vi "nD Nonlinear System Single Solution (Formula).vi"(7 "accuracy":dbl=1e-08 format="%0.2e", 8 "F(X)":string[](array[string]), 9 "X":string[](array[string]), 10 "Start":dbl[](array[numeric]) format="%0.2f", 11 "h":dbl=1e-08 format="%0.2e") -> (0 "error":i32, 1 "ticks":u32, 2 "f(Zeroes)":dbl[](array[numeric]) format="%0.2f", 3 "Zeroes":dbl[](array[numeric]) format="%0.2f")   [LabVIEW 2020, in "NI_Gmath.lvlib"]
doc: "Determines the solutions of nonlinear systems of equations in n dimensions beginning with a starting point in n dimensions. You must manually select the polymorphic instance to use."
uses:
  NI_Gmath.lvlib
  NI_AALBase.lvlib
panel:
  out "error message":string
  out "error text":string[](array[string])
  out "error code":i32[](array[numeric])
  # "Example:\n\n accuracy: 1E-8 \n h: 1E-8 \n Start: 1.0 and 0.0\n X: x and y\n F(X): sin(x+y) and cos(x-y)"
  # "error information"
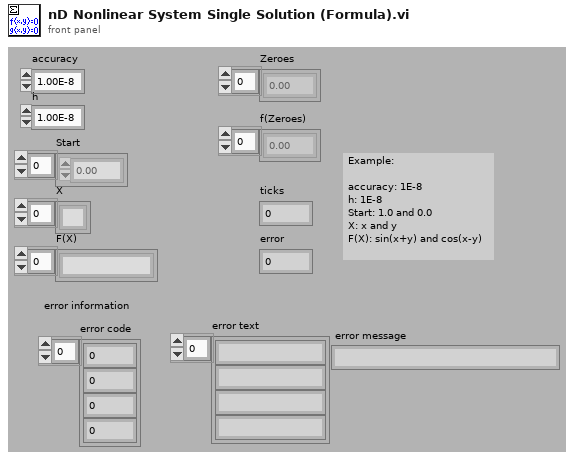
[diagram p1: front panel]
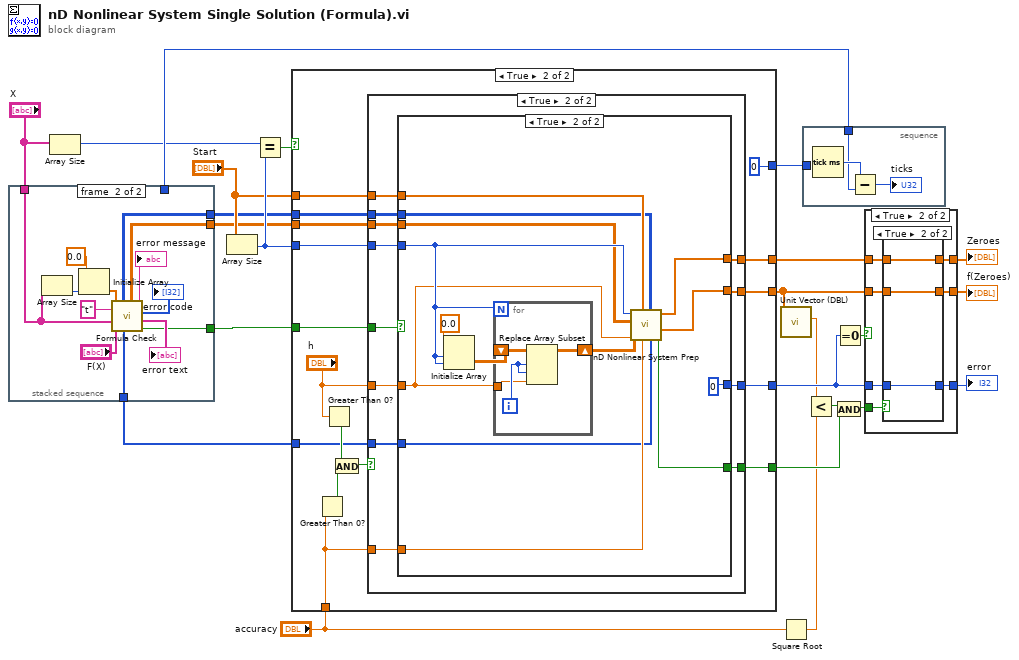
[diagram p0: block diagram]
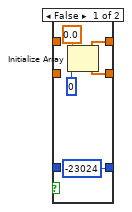
[diagram p3: hidden frame]
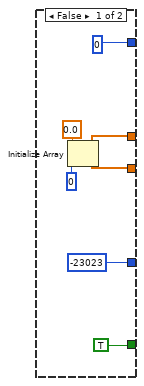
[diagram p4: hidden frame]
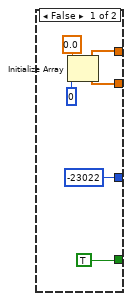
[diagram p5: hidden frame]
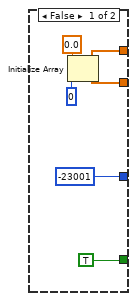
[diagram p6: hidden frame]
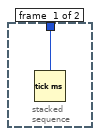
[diagram p7: hidden frame]
diagram:
  n1 = stacked-sequence {
    tunnel: [_ w30] -> w24
    tunnel: [w25 _] -> w22
    tunnel: "X" -> [_ w29]
    tunnel: [_ w28] -> w2
    tunnel: [_ w27] -> w3
    tunnel: [_ w26] -> w1
    frame #0 {
      n2 = Tick Count (ms)() -> (millisecond timer value=w25:u32)
    }
    frame #1 {
      n3 = Array Size(array=w29) -> (size(s)=w36:i32)
      n4 = Initialize Array(0.0, w36) -> (w38:dbl[])
      n5 = call "Formula Check.vi"("F(X,t)"="F(X)", "X"=w29, "time"="t", "X(0)"=w38) -> ("system error"=w30:bool, "error text"=→"error text":string[], "error"=→"error code":i32[], "error message"=→"error message":string, "result"=w28:dbl[][], "Variables"=w26:i32[], "Table"=w27:i32[][][])  [unwired: 1 out]
    }
  }
  n6 = Array Size(array="X") -> (size(s)=w18:i32)
  n7 = Array Size(array="Start") -> (size(s)=w21:i32)
  n8 = Equal?(x=w18, y=w21) -> (x = y?=w17:bool)
  n9 = case shown="True" w17 {
    tunnel: w21 -> [_ w60]
    tunnel: "Start" -> [_ w59]
    tunnel: [-23023 w58] -> w8
    tunnel: [w41 w57] -> w14
    tunnel: [w41 w56] -> w12
    tunnel: [0 0] -> w23
    tunnel: w24 -> [_ w55]
    tunnel: [TRUE w49] -> w10
    tunnel: "accuracy" -> [_ w48]
    tunnel: w3 -> [_ w47]
    tunnel: w2 -> [_ w46]
    tunnel: w1 -> [_ w45]
    frame False {
      n10 = Initialize Array(0.0, 0) -> (w41:dbl[])
    }
    frame True {
      n11 = Greater Than 0?(x=w48) -> (x > 0?=w53:bool)
      n12 = Greater Than 0?(x="h") -> (x > 0?=w52:bool)
      n13 = And(x=w52, y=w53) -> (x .and. y?=w51:bool)
      n14 = case shown="True" w51 {
        tunnel: w48 -> [_ w77]
        tunnel: "h" -> [_ w76]
        tunnel: w55 -> [_ w75]
        tunnel: [w63 w74] -> w56
        tunnel: [w63 w73] -> w57
        tunnel: [-23022 w72] -> w58
        tunnel: w59 -> [_ w71]
        tunnel: w60 -> [_ w70]
        tunnel: [TRUE w69] -> w49
        tunnel: w47 -> [_ w68]
        tunnel: w46 -> [_ w67]
        tunnel: w45 -> [_ w66]
        frame False {
          n15 = Initialize Array(0.0, 0) -> (w63:dbl[])
        }
        frame True {
          n16 = case shown="True" w75 {
            tunnel: [w79 w86] -> w74
            tunnel: [w79 w93] -> w73
            tunnel: [-23001 0] -> w72
            tunnel: w71 -> [_ w91]
            tunnel: w70 -> [_ w90]
            tunnel: w76 -> [_ w89]
            tunnel: w77 -> [_ w88]
            tunnel: [TRUE w87] -> w69
            tunnel: w68 -> [_ w85]
            tunnel: w67 -> [_ w84]
            tunnel: w66 -> [_ w83]
            frame False {
              n17 = Initialize Array(0.0, 0) -> (w79:dbl[])
            }
            frame True {
              n18 = Initialize Array(0.0, w90, w90) -> (w95:dbl[][])
              n19 = for {
                N: w90 -> [_]
                shift-right: [w99] -> w94
                shift-left: w95 -> [w100]
                tunnel: w89 -> [w97]
                i -> [w98]
                n20 = Replace Array Subset(array=w100, new element=w97, index (row)=w98, index (col)=w98) -> (w99:dbl[][])
              }
              n21 = call "nD Nonlinear System Prep.vi"("list of variables"=w83, "table"=w85, "accuracy"=w88, "Start"=w91, "h"=w89, "Diagonal h"=w94, "result"=w84, "length of Start"=w90) -> ("error"=w87:bool, "F(X)"=w93:dbl[], "Start new"=w86:dbl[])  [unwired: 1 out]
            }
          }
        }
      }
    }
  }
  n22 = call "Unit Vector (DBL).vi"("Input Vector"=w14) -> ("norm"=w4:dbl)  [unwired: 8 in, 2 out]
  n23 = Square Root(x="accuracy") -> (sqrt(x)=w5:dbl)
  n24 = stacked-sequence {
    tunnel: w22 -> [w102]
    tunnel: w23 -> [_]
    frame #0 {
      n25 = Tick Count (ms)() -> (millisecond timer value=w103:u32)
      n26 = Subtract(x=w103, y=w102) -> (x-y=→"ticks":u32)
    }
  }
  n27 = Less?(x=w4, y=w5) -> (x < y?=w13:bool)
  n28 = And(x=w13, y=w10) -> (x .and. y?=w9:bool)
  n29 = Equal To 0?(x=w8) -> (x = 0?=w7:bool)
  n30 = case shown="True" w7 {
    tunnel: [w106 w113] -> w11
    tunnel: w12 -> [w106 w112]
    tunnel: w9 -> [_ w111]
    tunnel: w14 -> [w105 w110]
    tunnel: [w104 w109] -> w15
    tunnel: w8 -> [w104 w108]
    tunnel: [w105 w107] -> w16
    frame False {
    }
    frame True {
      n31 = case shown="True" w111 {
        tunnel: w112 -> [_ w120]
        tunnel: [w115 w120] -> w113
        tunnel: w110 -> [_ w119]
        tunnel: [w115 w119] -> w107
        tunnel: w108 -> [_ w118]
        tunnel: [-23024 w118] -> w109
        frame False {
          n32 = Initialize Array(0.0, 0) -> (w115:dbl[])
        }
        frame True {
        }
      }
    }
  }
  "Zeroes" <- w11
  "f(Zeroes)" <- w16
  "error" <- w15
